vi "Image_Save.vi"(0 "Subfolder path":string, 5 "Subfolder Name":string, 7 "Timestamp":string, 9 "Image in":T1, 11 "error in":errorcluster, 12 "Camera":string) -> (4 "Image out":T1, 6 "path out":path, 15 "error out":errorcluster)   [LabVIEW 2019]
uses:
  <vilib>/vision/Image Controls.llb/IMAQ Image.ctl
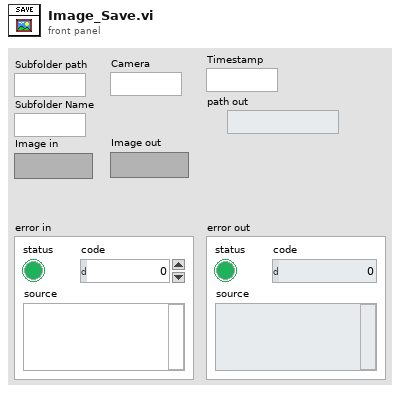
[diagram p1: front panel]
types:
  T1 = typedef "IMAQ Image.ctl" = refnum<image>
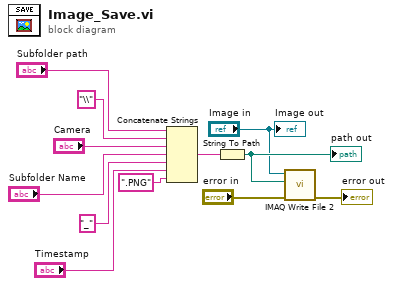
[diagram p0: block diagram]
diagram:
  n1 = Concatenate Strings("Subfolder path", "\\" ("string"), "Camera", "Subfolder Name", "_" ("string"), "Timestamp", ".PNG" ("string")) -> (w11:string)
  n2 = String To Path(string=w11) -> (path=w12:path)
  "path out" <- w12
  n3 = call-poly "IMAQ Write File 2"("error in (no error)"="error in", "File Path"=w12, "Image"="Image in") -> ("error out"=→"error out":errorcluster)  [unwired: 7 in, 1 out]
  "Image out" <- "Image in"
